vi "display_michelle_PKT_visjitter_stopadded_RandCont_PsuedoCO_TSLogFC2_forrecording.vi"() -> ()   [LabVIEW 2019]
uses:
  <vilib>/Analysis/Matrix/Datatypes/RealMatrix.ctl
  <vilib>/Utility/file.llb/Write Delimited Spreadsheet (DBL).vi
  <vilib>/Analysis/Matrix/NI_Matrix.lvlib
panel:
  out "lambda":dbl
  out "maxITI":dbl
  out "minITI":dbl
  out "goEXP":dbl
  out "meanITI":dbl
  out "Lag1":dbl
  out "TSLog":dbl[][](array[numeric])
  out "TSLog2":dbl[][](array[numeric])
  out "Initialtime":dbl
  out "Time Stamp":timestamp format="%<%H:%M:%S%4u>T"
  out "TSLog1":dbl[][](array[numeric])
  out "ArrayTemp3":T1
  out "StimID2":dbl
  out "Contrast":dbl
  out "TimeOutCounter":i32
  out "ElapsedTime_M":dbl
  out "Base_Contrast":dbl
  out "CurrentTrial":u32=1
  out "Jitter":dbl
  out "BaseITI":dbl
  out "VisStimDuration":dbl
  in  "Stop":bool
  out "Num trials":u32=204
  out "ISI Time":dbl
  out "Stim TS":dbl
  out "Output":dbl[][](array[numeric])
  out "Output frame":T1
  out "Array temp1":T1
  out "Elapsed Time":dbl
  out "Display":bool=TRUE
  out "Trial":u32=1
  out "reward":dbl[](array[numeric])
  out "stim_id":dbl[](array[numeric])
  out "stim_loaded":dbl
  out "Timings":dbl[](array[numeric])
  out "Stimuli Loaded?":bool
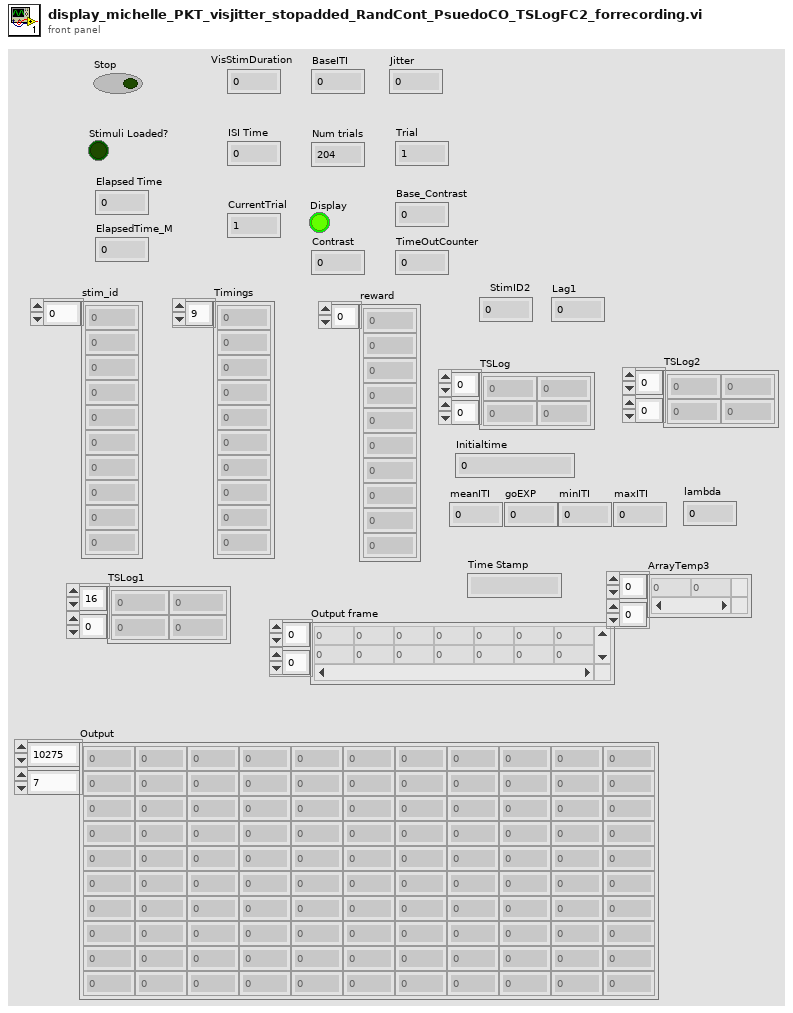
[diagram p1: front panel]
types:
  T1 = typedef "NI_Matrix.lvlib/RealMatrix.ctl" = dbl[][]
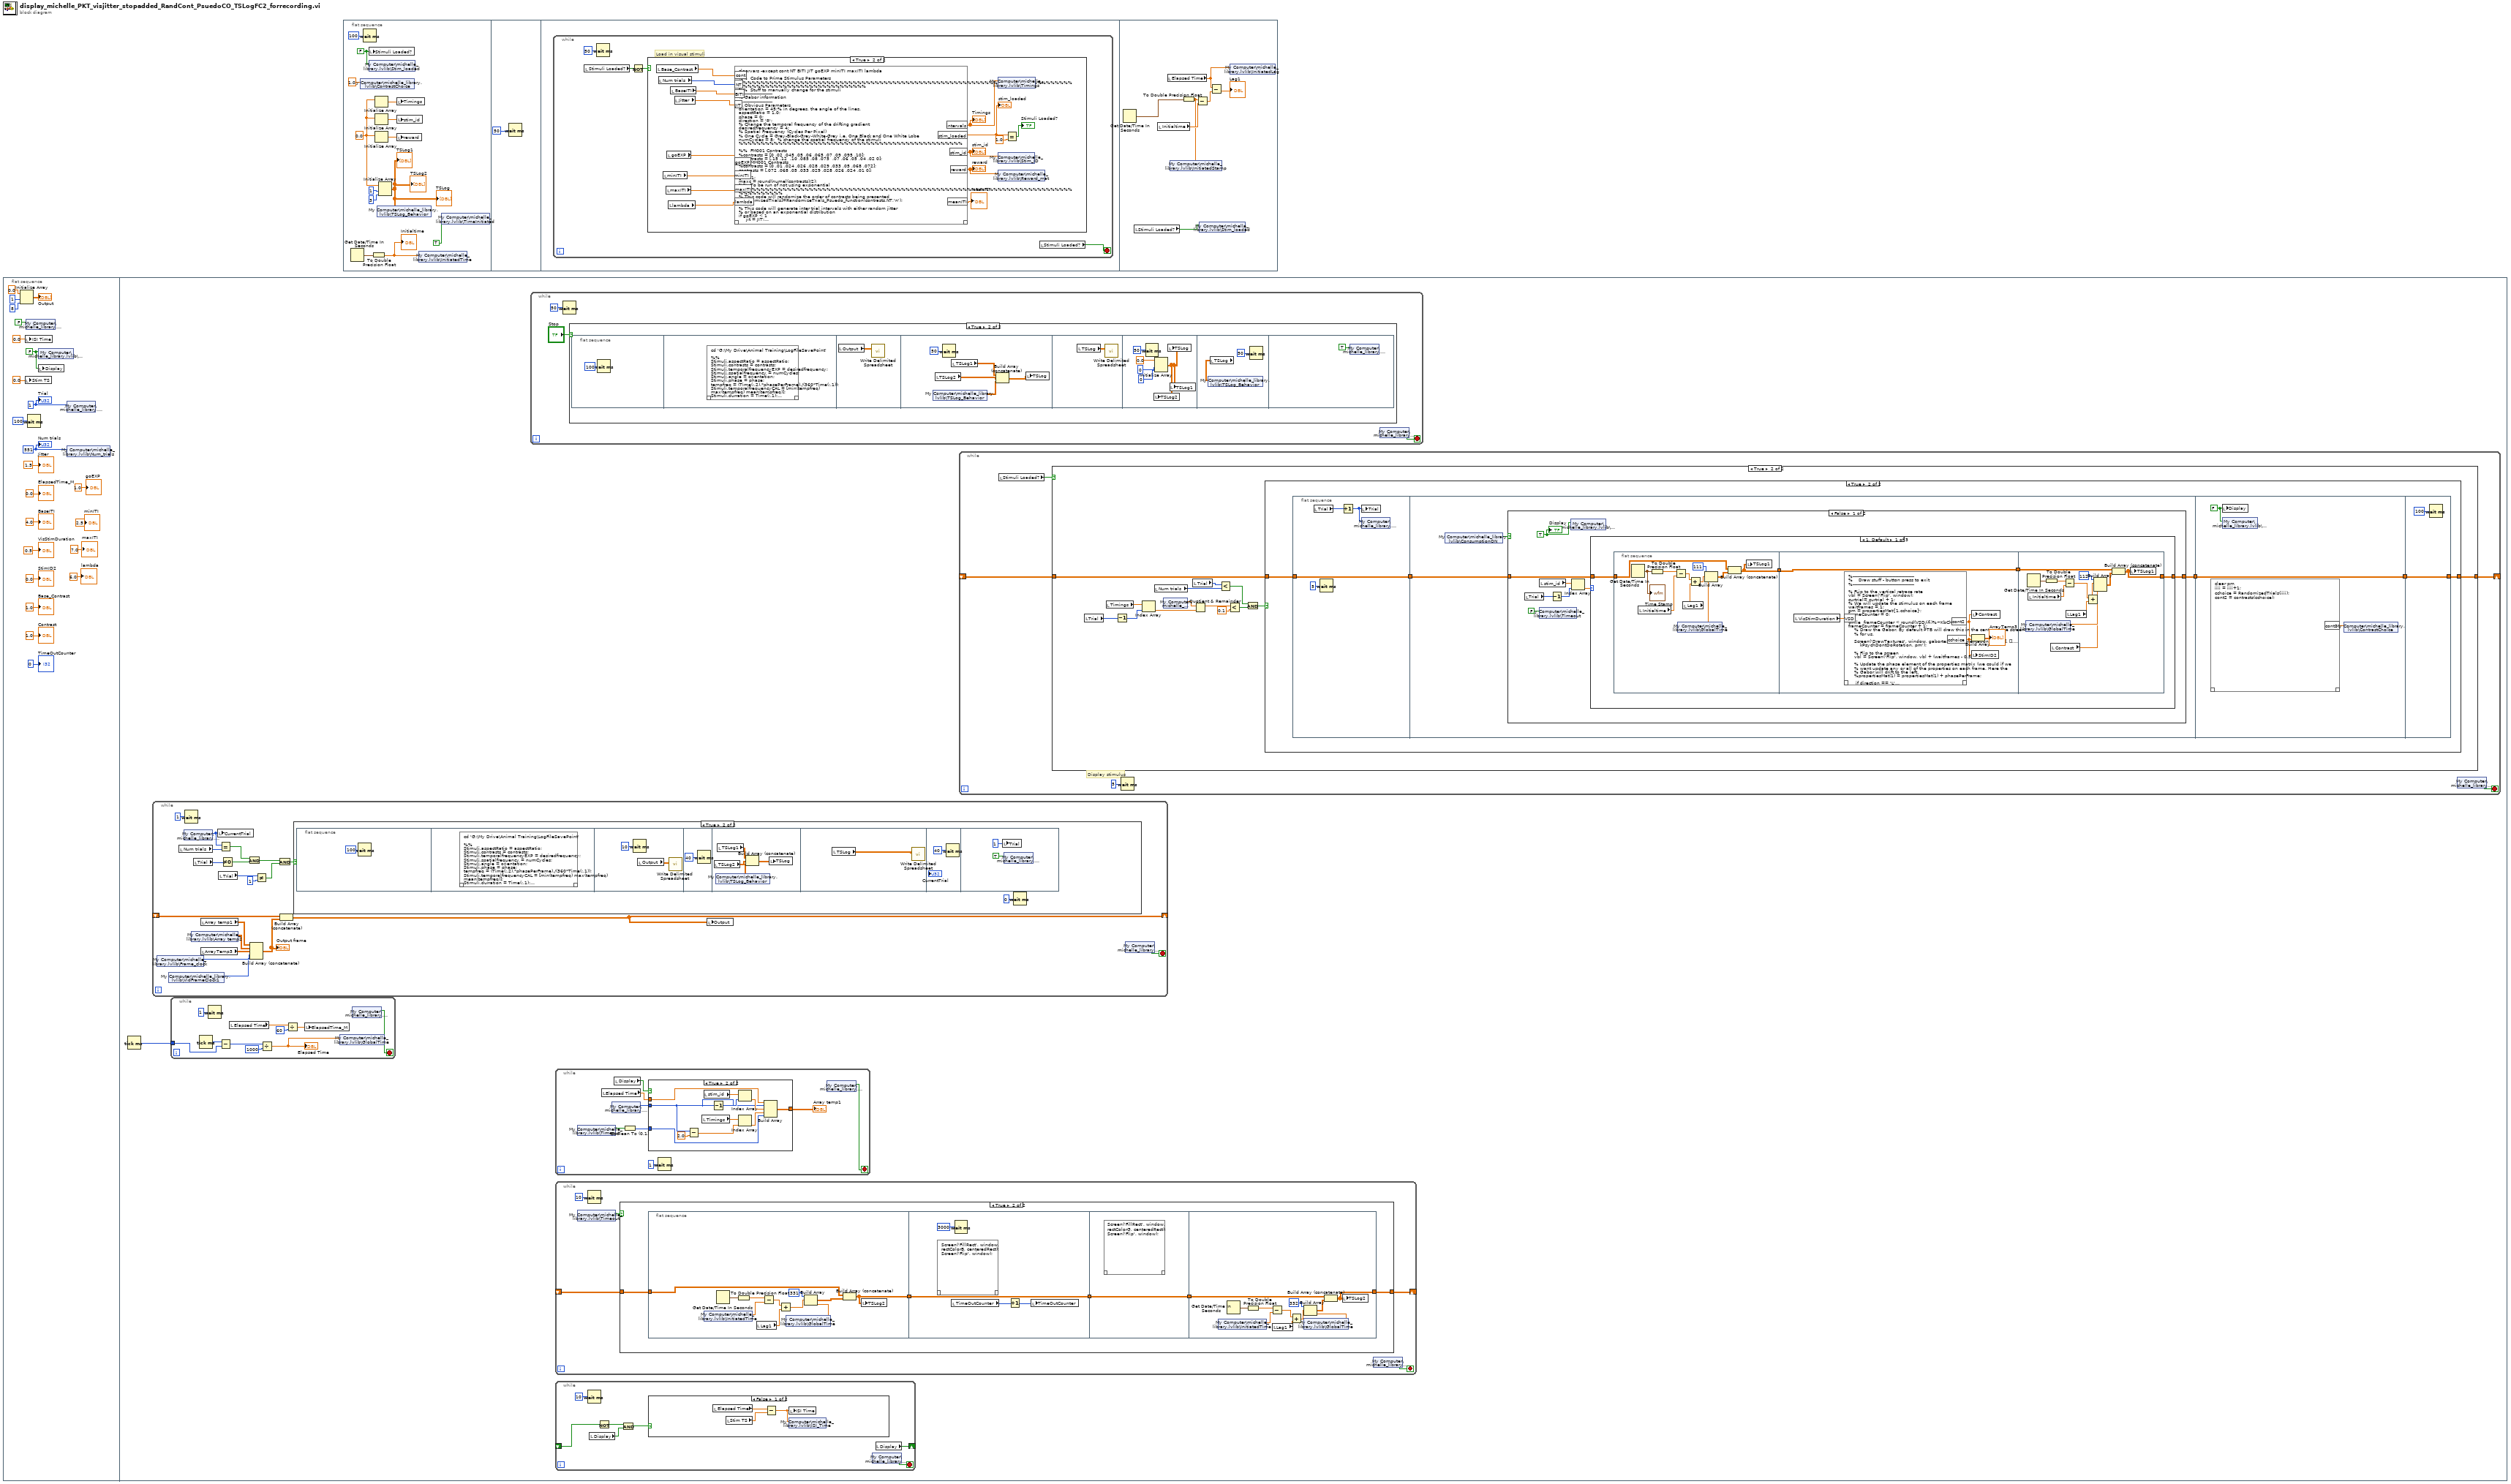
[diagram p0: block diagram]
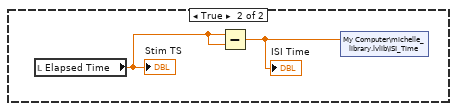
[diagram p5: hidden frame]
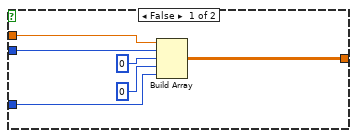
[diagram p6: hidden frame]
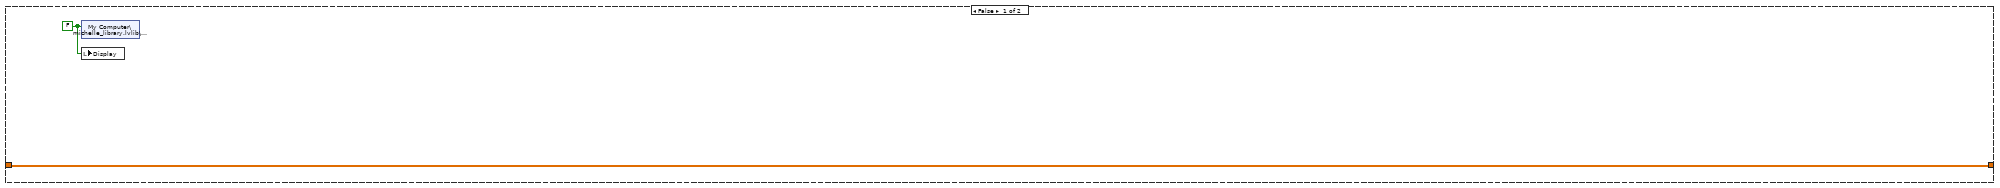
[diagram p9: hidden frame]
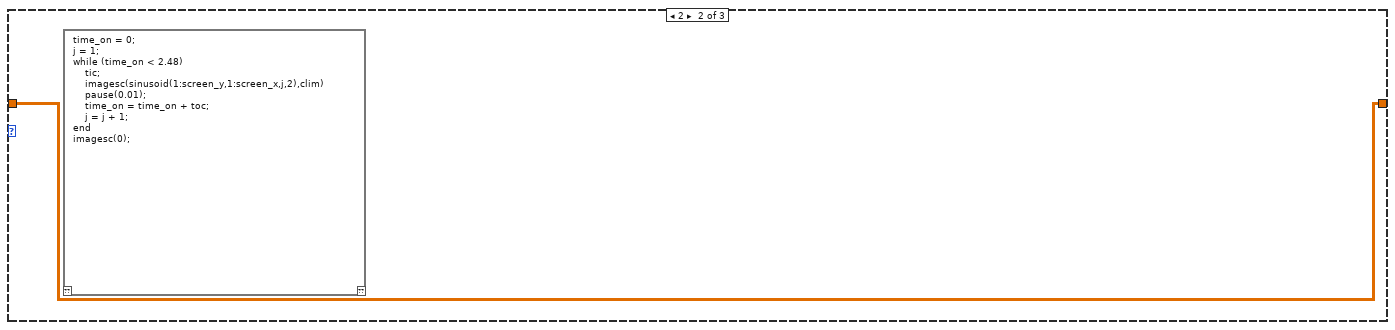
[diagram p10: hidden frame]
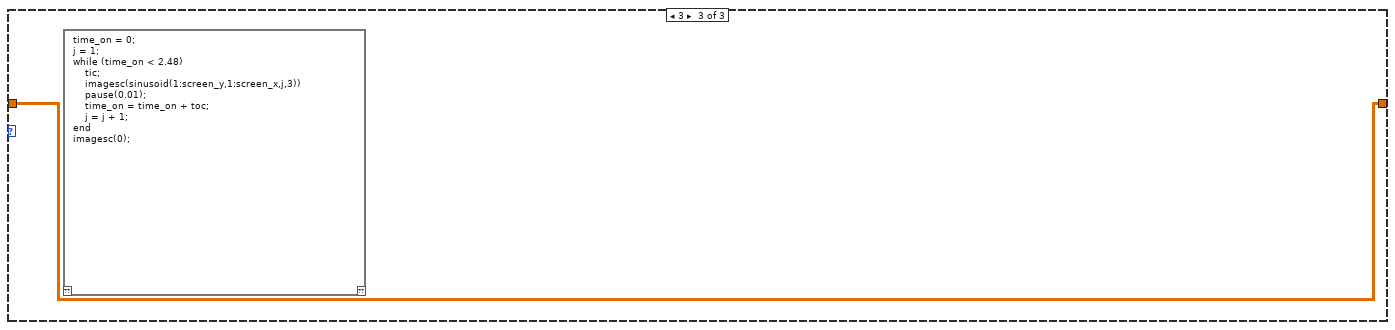
[diagram p11: hidden frame]
diagram:
  n1 = flat-sequence {
    frame #0 {
      w15 = u32 551
      w21 = FALSE ("Display")
      w23 = u32 1 ("Trial")
      n2 = Initialize Array(0.0 ("element"), 1 ("dimension size"), 8 ("dimension size")) -> (→"Output":dbl[][])
      n3 = local write "ISI Time"(0.0 ("ISI Time")) -> ()
      n4 = local write "Stim TS"(0.0 ("Stim TS")) -> ()
      n5 = shared-variable "My Computer\\michelle_library.lvlib\\Stop"(FALSE ("Stop")) -> ()  [unwired: 1 in, 1 out]
      n6 = Wait (ms)(milliseconds to wait=u32 100) -> ()  [unwired: 1 out]
      n7 = shared-variable "My Computer\\michelle_library.lvlib\\Display"(w21) -> ()  [unwired: 1 in, 1 out]
      n8 = local write "Display"(w21) -> ()
      n9 = shared-variable "My Computer\\michelle_library.lvlib\\Trial"(w23) -> ()  [unwired: 1 in, 1 out]
      n10 = shared-variable "My Computer\\michelle_library.lvlib\\Num_trials"(w15) -> ()  [unwired: 1 in, 1 out]
      "Trial" <- w23
      "Num trials" <- w15
      "VisStimDuration" <- 0.5
      "BaseITI" <- 4.0
      "Jitter" <- 1.5
      "Base_Contrast" <- 1.0
      "ElapsedTime_M" <- 0.0
      "TimeOutCounter" <- 0
      "Contrast" <- 1.0
      "StimID2" <- 0.0
      "goEXP" <- 1.0
      "minITI" <- 2.5
      "maxITI" <- 7.0
      "lambda" <- 6.0
    }
    frame #1 {
      n11 = Tick Count (ms)() -> (millisecond timer value=w24:u32)
      n12 = while {
        shift-right: [w145] -> _
        shift-left: _ -> [w146]
        stop <- w148 stop-if-true
        n13 = shared-variable "My Computer\\michelle_library.lvlib\\Frame_clock"() -> (w130:u32)  [unwired: 1 in, 1 out]
        n14 = shared-variable "My Computer\\michelle_library.lvlib\\VidFrameClock1"() -> (w129:u32)  [unwired: 1 in, 1 out]
        n15 = local read "Num trials"() -> (w141:u32)
        n16 = shared-variable "My Computer\\michelle_library.lvlib\\Trial"() -> (w132:u32)  [unwired: 1 in, 1 out]
        n17 = Wait (ms)(milliseconds to wait=u32 1) -> ()  [unwired: 1 out]
        n18 = shared-variable "My Computer\\michelle_library.lvlib\\Array temp2"() -> (w143:dbl[][])  [unwired: 1 in, 1 out]
        n19 = local read "Trial"() -> (w139:u32)
        n20 = local read "Array temp1"() -> (w144:T1)
        n21 = local read "ArrayTemp3"() -> (w131:T1)
        n22 = local write "CurrentTrial"(w132) -> ()
        n23 = local read "Trial"() -> (w138:u32)
        n24 = Equal?(x=w132, y=w141) -> (x = y?=w140:bool)
        n25 = Not Equal To 0?(x=w139) -> (x != 0?=w135:bool)
        n26 = And(x=w140, y=w135) -> (x .and. y?=w133:bool)
        n27 = Build Array (concatenate)(w144, w143, w131, w130, w129) -> (w142:T1)
        "Output frame" <- w142
        n28 = Not Equal?(x=w138, y=1) -> (x != y?=w137:bool)
        n29 = And(x=w133, y=w137) -> (x .and. y?=w134:bool)
        n30 = Build Array (concatenate) ("Build Matrix")(w146, w142) -> (w145:T1)
        n31 = case shown="True" w134 {
          frame False {
          }
          frame True {
            n32 = flat-sequence {
              frame #0 {
                n33 = Wait (ms)(milliseconds to wait=100) -> ()  [unwired: 1 out]
              }
              frame #1 {
                n34 = script code="cd 'G:\\My Drive\\Animal Training\\LogFileSavePoint'\n\n%%\nStimuli.aspectRatio = aspectRatio;\nStimuli.contrasts = contrasts;\nStimuli.temporalfrequencyEXP = desiredfrequency;\nStimuli.spatialfrequency = numCycles;\nStimuli.angle = orientation;\nStimuli.phase = phase;\ntempfreq = (Time(:,2).*phasePerFrame)./(360*Time(:,1)); \nStimuli.temporalfrequencyCAL = [min(tempfreq) max(tempfreq) mean(tempfreq)];\nStimuli.durration = Time(:,1);\nStimuli.frames = Time(:,2);\nStimuli.contrast = Time(:,3);\nStimuli.intervals = intervals;\nif goEXP == 0\n     int.type = 'jitter';\n     int.baseITI = BITI;\n     int.jitter = JIT;\nelseif goEXP == 1\n     int.type = 'exponential';\n     int.minITI = minITI;\n     int.maxITI = maxITI;\n     int.lambda = lambda;\nend\nStimuli.IntervalData = int;\n\n\nWindow.Xpixels = screenXpixels;\nWindow.Ypixels = screenYpixels;\nWindow.Xcenter = xCenter;\nWindow.Ycenter = yCenter;\nWindow.ifi = ifi;\nWindow.screen = screenNumber;\n\n%%\n[logname] = generatelogname();\n\nsave(logname,'Stimuli','Window');"() -> ()  [unwired: 1 in, 1 out]
              }
              frame #2 {
                n35 = Wait (ms)(milliseconds to wait=u32 10) -> ()  [unwired: 1 out]
                n36 = local read "Output"() -> (w152:dbl[][])
                n37 = call-poly <vilib>:"Write Delimited Spreadsheet.vi"("2D data"=w152) -> ()  [unwired: 13 in, 2 out]
              }
              frame #3 {
                n38 = Wait (ms)(milliseconds to wait=u32 40) -> ()  [unwired: 1 out]
              }
              frame #4 {
                n39 = local read "TSLog2"() -> (w157:dbl[][])
                n40 = shared-variable "My Computer\\michelle_library.lvlib\\TSLog_Behavior"() -> (w155:dbl[][])  [unwired: 1 in, 1 out]
                n41 = local read "TSLog1"() -> (w156:dbl[][])
                n42 = Build Array (concatenate) ("Build Matrix")(w156, w157, w155) -> (w154:T1)
                n43 = local write "TSLog"(w154) -> ()
              }
              frame #5 {
                n44 = local read "TSLog"() -> (w158:dbl[][])
                n45 = call-poly <vilib>:"Write Delimited Spreadsheet.vi"("2D data"=w158) -> ()  [unwired: 13 in, 2 out]
              }
              frame #6 {
                n46 = Wait (ms)(milliseconds to wait=u32 40) -> ()  [unwired: 1 out]
              }
              frame #7 {
                n47 = local write "Trial"(1) -> ()
                n48 = shared-variable "My Computer\\michelle_library.lvlib\\Stop"(TRUE) -> ()  [unwired: 1 in, 1 out]
              }
            }
            n49 = Wait (ms)(milliseconds to wait=0) -> ()  [unwired: 1 out]
          }
        }
        n50 = local write "Output"(w145) -> ()
        n51 = shared-variable "My Computer\\michelle_library.lvlib\\Stop"() -> (w148:bool)  [unwired: 1 in, 1 out]
      }
      n52 = while {
        tunnel: w24 -> [w126]
        stop <- w123 stop-if-true
        n53 = Tick Count (ms)() -> (millisecond timer value=w127:u32)
        n54 = Wait (ms)(milliseconds to wait=u32 1) -> ()  [unwired: 1 out]
        n55 = Subtract(x=w127, y=w126) -> (x-y=w124:u32)
        n56 = local read "Elapsed Time"() -> (w121:dbl)
        n57 = Divide(x=w124, y=u32 1000) -> (x/y=w119:dbl)
        "Elapsed Time" <- w119
        n58 = Divide(x=w121, y=60) -> (x/y=w120:dbl)
        n59 = local write "ElapsedTime_M"(w120) -> ()
        n60 = shared-variable "My Computer\\michelle_library.lvlib\\GlobalTime"(w119) -> ()  [unwired: 1 in, 1 out]
        n61 = shared-variable "My Computer\\michelle_library.lvlib\\Stop"() -> (w123:bool)  [unwired: 1 in, 1 out]
      }
      n62 = while {
        stop <- w27 stop-if-true
        n63 = Wait (ms)(milliseconds to wait=50) -> ()  [unwired: 1 out]
        n64 = case shown="True" "Stop" {
          frame False {
          }
          frame True {
            n65 = flat-sequence {
              frame #0 {
                n66 = Wait (ms)(milliseconds to wait=100) -> ()  [unwired: 1 out]
              }
              frame #1 {
                n67 = script code="cd 'G:\\My Drive\\Animal Training\\LogFileSavePoint'\n\n%%\nStimuli.aspectRatio = aspectRatio;\nStimuli.contrasts = contrasts;\nStimuli.temporalfrequencyEXP = desiredfrequency;\nStimuli.spatialfrequency = numCycles;\nStimuli.angle = orientation;\nStimuli.phase = phase;\ntempfreq = (Time(:,2).*phasePerFrame)./(360*Time(:,1)); \nStimuli.temporalfrequencyCAL = [min(tempfreq) max(tempfreq) mean(tempfreq)];\nStimuli.durration = Time(:,1);\nStimuli.frames = Time(:,2);\nStimuli.contrast = Time(:,3);\nStimuli.intervals = intervals;\nif goEXP == 0\n     int.type = 'jitter';\n     int.baseITI = BITI;\n     int.jitter = JIT;\nelseif goEXP == 1\n     int.type = 'exponential';\n     int.minITI = minITI;\n     int.maxITI = maxITI;\n     int.lambda = lambda;\nend\nStimuli.IntervalData = int;\n\n\nWindow.Xpixels = screenXpixels;\nWindow.Ypixels = screenYpixels;\nWindow.Xcenter = xCenter;\nWindow.Ycenter = yCenter;\nWindow.ifi = ifi;\nWindow.screen = screenNumber;\n\n%%\n[logname] = generatelogname();\n\nsave(logname,'Stimuli','Window');"() -> ()  [unwired: 1 in, 1 out]
              }
              frame #2 {
                n68 = local read "Output"() -> (w29:dbl[][])
                n69 = call-poly <vilib>:"Write Delimited Spreadsheet.vi"("2D data"=w29) -> ()  [unwired: 13 in, 2 out]
              }
              frame #3 {
                n70 = shared-variable "My Computer\\michelle_library.lvlib\\TSLog_Behavior"() -> (w30:dbl[][])  [unwired: 1 in, 1 out]
                n71 = local read "TSLog2"() -> (w33:dbl[][])
                n72 = Wait (ms)(milliseconds to wait=50) -> ()  [unwired: 1 out]
                n73 = local read "TSLog1"() -> (w32:dbl[][])
                n74 = Build Array (concatenate) ("Build Matrix")(w32, w33, w30) -> (w31:T1)
                n75 = local write "TSLog"(w31) -> ()
              }
              frame #4 {
                n76 = local read "TSLog"() -> (w35:dbl[][])
                n77 = call-poly <vilib>:"Write Delimited Spreadsheet.vi"("2D data"=w35) -> ()  [unwired: 13 in, 2 out]
              }
              frame #5 {
                n78 = Wait (ms)(milliseconds to wait=50) -> ()  [unwired: 1 out]
                n79 = Initialize Array(0.0, 0, 0) -> (w37:dbl[][])
                n80 = local write "TSLog2"(w37) -> ()
                n81 = local write "TSLog"(w37) -> ()
                n82 = local write "TSLog1"(w37) -> ()
              }
              frame #6 {
                n83 = local read "TSLog"() -> (w42:dbl[][])
                n84 = shared-variable "My Computer\\michelle_library.lvlib\\TSLog_Behavior"(w42) -> ()  [unwired: 1 in, 1 out]
                n85 = Wait (ms)(milliseconds to wait=50) -> ()  [unwired: 1 out]
              }
              frame #7 {
                n86 = shared-variable "My Computer\\michelle_library.lvlib\\Stop"(TRUE) -> ()  [unwired: 1 in, 1 out]
              }
            }
          }
        }
        n87 = shared-variable "My Computer\\michelle_library.lvlib\\Stop"() -> (w27:bool)  [unwired: 1 in, 1 out]
      }
      n88 = while {
        stop <- w96 stop-if-true
        n89 = shared-variable "My Computer\\michelle_library.lvlib\\Timeout"() -> (w94:bool)  [unwired: 1 in, 1 out]
        n90 = local read "Elapsed Time"() -> (w100:dbl)
        n91 = shared-variable "My Computer\\michelle_library.lvlib\\Trial"() -> (w98:u32)  [unwired: 1 in, 1 out]
        n92 = local read "Display"() -> (w97:bool)
        n93 = Boolean To (0,1)(Boolean=w94) -> (0, 1=w95:i16)
        n94 = case shown="True" w97 {
          tunnel: w98 -> [w106 w109]
          tunnel: w100 -> [w107 w116]
          tunnel: [w105 w117] -> w99
          tunnel: w95 -> [w102 w111]
          frame False {
            n95 = Build Array(w107, w106, u32 0 ("milliseconds to wait"), 0, w102) -> (w105:T1)
          }
          frame True {
            n96 = Subtract(x=w109, y=2.0) -> (x-y=w108:dbl)
            n97 = local read "Timings"() -> (w114:dbl[])
            n98 = local read "stim_id"() -> (w118:dbl[])
            n99 = Decrement(x=w109) -> (x-1=w113:u32)
            n100 = Index Array(array=w118, index=w113) -> (element=w115:dbl)
            n101 = Index Array(array=w114, index=w108) -> (element=w112:dbl)
            n102 = Build Array(w116, w109, w115, w112, w111) -> (w117:T1)
          }
        }
        "Array temp1" <- w99
        n103 = Wait (ms)(milliseconds to wait=u32 1) -> ()  [unwired: 1 out]
        n104 = shared-variable "My Computer\\michelle_library.lvlib\\Stop"() -> (w96:bool)  [unwired: 1 in, 1 out]
      }
      n105 = while {
        shift-right: [w44] -> _
        shift-left: _ -> [w45]
        stop <- w48 stop-if-true
        n106 = shared-variable "My Computer\\michelle_library.lvlib\\Timeout"() -> (w46:bool)  [unwired: 1 in, 1 out]
        n107 = Wait (ms)(milliseconds to wait=u32 10) -> ()  [unwired: 1 out]
        n108 = case shown="True" w46 {
          tunnel: w45 -> [w49 w54]
          tunnel: [w49 w53] -> w44
          frame False {
          }
          frame True {
            n109 = flat-sequence {
              tunnel: w54 -> [w60]
              tunnel: [w59] -> w51
              tunnel: [w66] -> w52
              tunnel: w51 -> [w66]
              tunnel: w52 -> [w70]
              tunnel: [w70] -> w50
              tunnel: [w75] -> w53
              tunnel: w50 -> [w76]
              frame #0 {
                n110 = shared-variable "My Computer\\michelle_library.lvlib\\InitiatedTime"() -> (w63:dbl)  [unwired: 1 in, 1 out]
                n111 = Get Date/Time In Seconds() -> (seconds since 1Jan1904=w65:timestamp)
                n112 = To Double Precision Float(number=w65) -> (double precision float=w64:dbl)
                n113 = local read "Lag1"() -> (w56:dbl)
                n114 = Subtract(x=w64, y=w63) -> (x-y=w57:dbl)
                n115 = Add(x=w57, y=w56) -> (x+y=w58:dbl)
                n116 = shared-variable "My Computer\\michelle_library.lvlib\\GlobalTime"() -> (w55:dbl)  [unwired: 1 in, 1 out]
                n117 = Build Array(331, w58, w55) -> (w62:T1)
                n118 = Build Array (concatenate) ("Build Matrix")(w60, w62) -> (w59:T1)
                n119 = local write "TSLog2"(w59) -> ()
              }
              frame #1 {
                n120 = script code="Screen('FillRect', window, rectColorB, centeredRect);\nScreen('Flip', window);"() -> ()  [unwired: 1 in, 1 out]
                n121 = local read "TimeOutCounter"() -> (w68:i32)
                n122 = Wait (ms)(milliseconds to wait=u32 3000) -> ()  [unwired: 1 out]
                n123 = Increment(x=w68) -> (x+1=w67:i32)
                n124 = local write "TimeOutCounter"(w67) -> ()
              }
              frame #2 {
                n125 = script code="Screen('FillRect', window, rectColorG, centeredRect);\nScreen('Flip', window);"() -> ()  [unwired: 1 in, 1 out]
              }
              frame #3 {
                n126 = shared-variable "My Computer\\michelle_library.lvlib\\InitiatedTime"() -> (w81:dbl)  [unwired: 1 in, 1 out]
                n127 = Get Date/Time In Seconds() -> (seconds since 1Jan1904=w79:timestamp)
                n128 = To Double Precision Float(number=w79) -> (double precision float=w80:dbl)
                n129 = Subtract(x=w80, y=w81) -> (x-y=w73:dbl)
                n130 = local read "Lag1"() -> (w72:dbl)
                n131 = Add(x=w73, y=w72) -> (x+y=w74:dbl)
                n132 = shared-variable "My Computer\\michelle_library.lvlib\\GlobalTime"() -> (w71:dbl)  [unwired: 1 in, 1 out]
                n133 = Build Array(332, w74, w71) -> (w77:T1)
                n134 = Build Array (concatenate) ("Build Matrix")(w76, w77) -> (w75:T1)
                n135 = local write "TSLog2"(w75) -> ()
              }
            }
          }
        }
        n136 = shared-variable "My Computer\\michelle_library.lvlib\\Stop"() -> (w48:bool)  [unwired: 1 in, 1 out]
      }
      n137 = while {
        shift-right: [w86] -> _
        shift-left: _ -> [w85]
        stop <- w88 stop-if-true
        n138 = Wait (ms)(milliseconds to wait=u32 10) -> ()  [unwired: 1 out]
        n139 = local read "Display"() -> (w83:bool)
        n140 = Not(x=w85) -> (.not. x?=w84:bool)
        n141 = And(x=w84, y=w83) -> (x .and. y?=w82:bool)
        n142 = case shown="False" w82 {
          frame False {
            n143 = local read "Elapsed Time"() -> (w89:dbl)
            n144 = local read "Stim TS"() -> (w91:dbl)
            n145 = Subtract(x=w89, y=w91) -> (x-y=w90:dbl)
            n146 = local write "ISI Time"(w90) -> ()
            n147 = shared-variable "My Computer\\michelle_library.lvlib\\ISI_Time"(w90) -> ()  [unwired: 1 in, 1 out]
          }
          frame True {
            n148 = local read "Elapsed Time"() -> (w92:dbl)
            "Stim TS" <- w92
            n149 = Subtract(x=w92, y=w92) -> (x-y=w93:dbl)
            "ISI Time" <- w93
            n150 = shared-variable "My Computer\\michelle_library.lvlib\\ISI_Time"(w93) -> ()  [unwired: 1 in, 1 out]
          }
        }
        n151 = shared-variable "My Computer\\michelle_library.lvlib\\Stop"() -> (w88:bool)  [unwired: 1 in, 1 out]
        n152 = local read "Display"() -> (w86:bool)
      }
      n153 = while {
        shift-right: [w162] -> _
        shift-left: _ -> [w163]
        stop <- w165 stop-if-true
        # "Display stimulus"
        n154 = local read "Stimuli Loaded?"() -> (w164:bool)
        n155 = case shown="True" w164 {
          tunnel: w163 -> [w167 w169]
          tunnel: [w167 w168] -> w162
          frame False {
          }
          frame True {
            n156 = local read "Trial"() -> (w170:u32)
            n157 = local read "Timings"() -> (w179:dbl[])
            n158 = Decrement(x=w170) -> (x-1=w171:u32)
            n159 = Index Array(array=w179, index=w171) -> (element=w178:dbl)
            n160 = local read "Num trials"() -> (w174:u32)
            n161 = shared-variable "My Computer\\michelle_library.lvlib\\ISI"() -> (w173:dbl)  [unwired: 1 in, 1 out]
            n162 = local read "Trial"() -> (w177:u32)
            n163 = Quotient & Remainder(x=w173, y=w178) -> (x-y*floor(x/y)=w181:dbl)  [unwired: 1 out]
            n164 = Less?(x=w177, y=w174) -> (x < y?=w176:bool)
            n165 = Less?(x=w181, y=0.1) -> (x < y?=w175:bool)
            n166 = And(x=w176, y=w175) -> (x .and. y?=w172:bool)
            n167 = case shown="True" w172 {
              tunnel: w169 -> [w182 w187]
              tunnel: [w182 w186] -> w168
              frame False {
                w183 = FALSE ("Display")
                n168 = shared-variable "My Computer\\michelle_library.lvlib\\Display"(w183) -> ()  [unwired: 1 in, 1 out]
                n169 = local write "Display"(w183) -> ()
              }
              frame True {
                n170 = flat-sequence {
                  tunnel: [w189] -> w188
                  tunnel: w187 -> [w189]
                  tunnel: w188 -> [w194]
                  tunnel: [w193] -> w184
                  tunnel: [w239] -> w185
                  tunnel: w184 -> [w239]
                  tunnel: [w242] -> w186
                  tunnel: w185 -> [w242]
                  frame #0 {
                    n171 = local read "Trial"() -> (w192:u32)
                    n172 = Wait (ms)(milliseconds to wait=u32 5) -> ()  [unwired: 1 out]
                    n173 = Increment(x=w192) -> (x+1=w191:u32)
                    n174 = local write "Trial"(w191) -> ()
                    n175 = shared-variable "My Computer\\michelle_library.lvlib\\Trial"(w191) -> ()  [unwired: 1 in, 1 out]
                  }
                  frame #1 {
                    n176 = shared-variable "My Computer\\michelle_library.lvlib\\ConsumptionON"() -> (w195:bool)  [unwired: 1 in, 1 out]
                    n177 = case shown="False" w195 {
                      tunnel: w194 -> [w197 w238]
                      tunnel: [w196 w238] -> w193
                      frame False {
                        w198 = TRUE ("Boolean")
                        n178 = local read "Trial"() -> (w201:u32)
                        n179 = shared-variable "My Computer\\michelle_library.lvlib\\Timeout"(FALSE) -> ()  [unwired: 1 in, 1 out]
                        n180 = local read "stim_id"() -> (w203:dbl[])
                        n181 = Decrement(x=w201) -> (x-1=w200:u32)
                        n182 = shared-variable "My Computer\\michelle_library.lvlib\\Display"(w198) -> ()  [unwired: 1 in, 1 out]
                        n183 = Index Array(array=w203, index=w200) -> (element=w202:dbl)
                        n184 = case shown="1, Default" w202 {
                          tunnel: w197 -> [w207 w236 w237]
                          tunnel: [w206 w236 w237] -> w196
                          frame 1, Default {
                            n185 = flat-sequence {
                              tunnel: w207 -> [w217]
                              tunnel: [w216] -> w205
                              tunnel: w205 -> [w219]
                              tunnel: [w219] -> w204
                              tunnel: [w234] -> w206
                              tunnel: w204 -> [w233]
                              frame #0 {
                                n186 = Get Date/Time In Seconds() -> (seconds since 1Jan1904=w214:timestamp)
                                "Time Stamp" <- w214
                                n187 = local read "Initialtime"() -> (w212:dbl)
                                n188 = To Double Precision Float(number=w214) -> (double precision float=w213:dbl)
                                n189 = Subtract(x=w213, y=w212) -> (x-y=w210:dbl)
                                n190 = shared-variable "My Computer\\michelle_library.lvlib\\GlobalTime"() -> (w208:dbl)  [unwired: 1 in, 1 out]
                                n191 = local read "Lag1"() -> (w211:dbl)
                                n192 = Add(x=w210, y=w211) -> (x+y=w209:dbl)
                                n193 = Build Array(111, w209, w208) -> (w215:T1)
                                n194 = Build Array (concatenate) ("Build Matrix")(w217, w215) -> (w216:T1)
                                n195 = local write "TSLog1"(w216) -> ()
                              }
                              frame #1 {
                                n196 = local read "VisStimDuration"() -> (w221:dbl)
                                n197 = script code="%------------------------------------------\n%    Draw stuff - button press to exit\n%------------------------------------------\n\n% FLip to the vertical retrace rate\nvbl = Screen('Flip', window);\ncurtrial= curtrial + 1;\n% We will update the stimulus on each frame\nwaitframes = 1;\npm = propertiesMat{1,cchoice};\nframeCounter = 0;\ntic\nwhile  frameCounter < round(VSD/ifi)%~KbCheck\nframeCounter = frameCounter + 1;\n    % Draw the Gabor. By default PTB will draw this in the center of the screen\n    % for us.\n   \n    Screen('DrawTextures', window, gabortex, [], [], orientation, [], [], [], [],...\n        kPsychDontDoRotation, pm');\n\n    % Flip to the screen\n    vbl = Screen('Flip', window, vbl + (waitframes - 0.5) * ifi);\n\n    % Update the phase element of the properties matrix (we could if we\n    % want update any or all of the properties on each frame. Here the\n    % Gabor will drift to the left.\n    %propertiesMat(1) = propertiesMat(1) + phasePerFrame;\n \n     if direction == 'L'\n          pm(1) = pm(1) + phasePerFrame;\n     elseif direction =='R'\n          pm(1) = pm(1) - phasePerFrame;\n     end\n\nend\nTime(curtrial,1) = toc;\nTime(curtrial,2) = frameCounter;\nTime(curtrial,3) = pm(4);\nvbl = Screen('Flip', window);"("VSD"=w221) -> ("cont2"=w223:dbl, "cchoice"=w222:dbl)  [unwired: 1 in, 1 out]
                                n198 = local write "Contrast"(w223) -> ()
                                n199 = Build Array(w223, w222) -> (→"ArrayTemp3":T1)
                                n200 = local write "StimID2"(w222) -> ()
                              }
                              frame #2 {
                                n201 = shared-variable "My Computer\\michelle_library.lvlib\\GlobalTime"() -> (w225:dbl)  [unwired: 1 in, 1 out]
                                n202 = Get Date/Time In Seconds() -> (seconds since 1Jan1904=w231:timestamp)
                                n203 = local read "Initialtime"() -> (w230:dbl)
                                n204 = To Double Precision Float(number=w231) -> (double precision float=w229:dbl)
                                n205 = local read "Contrast"() -> (w224:dbl)
                                n206 = Subtract(x=w229, y=w230) -> (x-y=w228:dbl)
                                n207 = local read "Lag1"() -> (w226:dbl)
                                n208 = Add(x=w228, y=w226) -> (x+y=w227:dbl)
                                n209 = Build Array(112, w227, w225, w224) -> (w235:T1)
                                n210 = Build Array (concatenate) ("Build Matrix")(w233, w235) -> (w234:T1)
                                n211 = local write "TSLog1"(w234) -> ()
                              }
                            }
                          }
                          frame 2 {
                            n212 = script code="time_on = 0;\nj = 1;\nwhile (time_on < 2.48)\n    tic;\n    imagesc(sinusoid(1:screen_y,1:screen_x,j,2),clim)\n    pause(0.01);\n    time_on = time_on + toc;\n    j = j + 1;\nend\nimagesc(0);"() -> ()  [unwired: 1 in, 1 out]
                          }
                          frame 3 {
                            n213 = script code="time_on = 0;\nj = 1;\nwhile (time_on < 2.48)\n    tic;\n    imagesc(sinusoid(1:screen_y,1:screen_x,j,3))\n    pause(0.01);\n    time_on = time_on + toc;\n    j = j + 1;\nend\nimagesc(0);"() -> ()  [unwired: 1 in, 1 out]
                          }
                        }
                        "Display" <- w198
                      }
                      frame True {
                      }
                    }
                  }
                  frame #2 {
                    w241 = FALSE ("Display")
                    n214 = script code="clear pm\niiii = iiii+1;\ncchoice = RandomizedTrials(iiii);\ncont2 = contrasts(cchoice);"() -> ("cont2"=w240:dbl)  [unwired: 1 in, 1 out]
                    n215 = local write "Display"(w241) -> ()
                    n216 = shared-variable "My Computer\\michelle_library.lvlib\\Display"(w241) -> ()  [unwired: 1 in, 1 out]
                    n217 = shared-variable "My Computer\\michelle_library.lvlib\\ContrastChoice"(w240) -> ()  [unwired: 1 in, 1 out]
                  }
                  frame #3 {
                    n218 = Wait (ms)(milliseconds to wait=u32 100) -> ()  [unwired: 1 out]
                  }
                }
              }
            }
          }
        }
        n219 = Wait (ms)(milliseconds to wait=u32 5) -> ()  [unwired: 1 out]
        n220 = shared-variable "My Computer\\michelle_library.lvlib\\Stop"() -> (w165:bool)  [unwired: 1 in, 1 out]
      }
    }
  }
  n221 = flat-sequence {
    frame #0 {
      w250 = 0.0 ("element")
      w252 = FALSE ("Stimuli Loaded?")
      n222 = Get Date/Time In Seconds() -> (seconds since 1Jan1904=w247:timestamp)
      n223 = shared-variable "My Computer\\michelle_library.lvlib\\ContrastChoice"(1.0) -> ()  [unwired: 1 in, 1 out]
      n224 = Wait (ms)(milliseconds to wait=u32 100) -> ()  [unwired: 1 out]
      n225 = local write "Stimuli Loaded?"(w252) -> ()
      n226 = shared-variable "My Computer\\michelle_library.lvlib\\Stim_loaded"(w252) -> ()  [unwired: 1 in, 1 out]
      n227 = To Double Precision Float(number=w247) -> (double precision float=w246:dbl)
      "Initialtime" <- w246
      n228 = Initialize Array(w250) -> (w255:dbl[])  [unwired: 1 in]
      n229 = Initialize Array(w250) -> (w254:dbl[])  [unwired: 1 in]
      n230 = Initialize Array(w250) -> (w253:dbl[])  [unwired: 1 in]
      n231 = Initialize Array(w250, 1, 3) -> (w244:dbl[][])
      "TSLog1" <- w244
      "TSLog2" <- w244
      "TSLog" <- w244
      n232 = shared-variable "My Computer\\michelle_library.lvlib\\TSLog_Behavior"(w244) -> ()  [unwired: 1 in, 1 out]
      n233 = local write "Timings"(w255) -> ()
      n234 = local write "stim_id"(w254) -> ()
      n235 = local write "reward"(w253) -> ()
      n236 = shared-variable "My Computer\\michelle_library.lvlib\\InitiatedTime"(w246) -> ()  [unwired: 1 in, 1 out]
      n237 = shared-variable "My Computer\\michelle_library.lvlib\\TimeInitiated"(TRUE) -> ()  [unwired: 1 in, 1 out]
    }
    frame #1 {
      n238 = Wait (ms)(milliseconds to wait=u32 50) -> ()  [unwired: 1 out]
    }
    frame #2 {
      n239 = while {
        stop <- w258 stop-if-true
        # "Load in visual stimuli"
        n240 = local read "Stimuli Loaded?"() -> (w260:bool)
        n241 = Wait (ms)(milliseconds to wait=u32 50) -> ()  [unwired: 1 out]
        n242 = Not(x=w260) -> (.not. x?=w259:bool)
        n243 = case shown="True" w259 {
          frame False {
          }
          frame True {
            n244 = local read "Base_Contrast"() -> (w268:dbl)
            n245 = local read "Num trials"() -> (w271:u32)
            n246 = local read "minITI"() -> (w264:dbl)
            n247 = local read "maxITI"() -> (w263:dbl)
            n248 = local read "goEXP"() -> (w265:dbl)
            n249 = local read "lambda"() -> (w262:dbl)
            n250 = local read "BaseITI"() -> (w270:dbl)
            n251 = local read "Jitter"() -> (w269:dbl)
            n252 = script code="clearvars -except cont NT BITI JIT goEXP minITI maxITI lambda\n\n%%  Code to Prime Stimulus Parameters\n%%%%%%%%%%%%%%%%%%%%%%%%%%%%%%%%%%%%%%%%%%%%%%%%%%%%%%%%%%%%%%%%%%%%%%%%%%%%%%%%%%%%%%%%%%%%%%%%%%%%%%%%%\n%%  Stuff to manually change for the stimuli\n%--------------------\n% Gabor information\n%--------------------\n% Obvious Parameters\norientation = 45;% in degrees, the angle of the lines.\naspectRatio = 1.0;\nphase = 0;\ndirection = 'R';\n% Change the temporal frequency of the drifting gradient\ndesiredfrequency = 4;\n% Spatial Frequency (Cycles Per Pixel)\n% One Cycle = Grey-Black-Grey-White-Grey i.e. One Black and One White Lobe\nnumCycles = 8;  % change the spatial frequency of the stimuli\n%%%%%%%%%%%%%%%%%%%%%%%%%%%%%%%%%%%%%%%%%%%%%%%%%%%\n\n%%  FM001 Contrasts\n%contrasts = [0 .02 .045 .05 .06 .065 .07 .09 .095 .10];\n%contrasts = [.15 .12  .10 .085 .08 .075  .07 .06 .05 .04 .02 0];\n%%  MM001 Contrasts\n%contrasts = [0 .01 .024 .026 .028 .029 .033 .05 .068 .072];\ncontrasts = [.072 .068 .05 .033 .029 .028 .026 .024 .01 0];\n\ngo = 1;\nmaxc = round(numel(contrasts)/2);\n%%  To be run of not using exponential\n%%%%%%%%%%%%%%%%%%%%%%%%%%%%%%%%%%%%%%%%%%%%%%%%%%%%%%%%%%%%%%%%%%%%%%%%%%%%%%%%%%%%%%\n% This code will randomize the order of contrasts being presented\n[RandomizedTrials]=RandomizeTrials_Psuedo_function(contrasts,NT,'n');\n\n% This code will generate inter trial intervals with either random jitter\n% or based on an exponential distribution\nif goEXP < 1\n     jit = JIT;\n     jitter = rand(1,NT);\n     jitter = 2*jit*(jitter- .5);\n     ITIbase = BITI;\n     intervals = [ones(1,NT)*ITIbase];\n     intervals = intervals + jitter;\nelseif goEXP > 0\n     intervals = exponentialITI(1/lambda, minITI, maxITI, NT);\nend\n\n%%  Prep the stimulus presentation software\n%%%%%%%%%%%%%%%%%%%%%%%%%%%%%%%%%%%%%%%%%%%%%%%%%%%%%%%%%%%%%%%%%%%%%%%%%%%\nScreen('Preference', 'SkipSyncTests', 1);\nsca;\nclose all;\n% Setup PTB with some default values\nPsychDefaultSetup(2);\n% Set the screen number to the external secondary monitor if there is one connected\nscreenNumber = max(Screen('Screens'));\n\n% Define black, white and grey\nwhite = WhiteIndex(screenNumber);\nblack = BlackIndex(screenNumber);\ngrey = white / 2;\n\n% Open the screen & define it's dimensions\n[window, windowRect] = PsychImaging('OpenWindow', screenNumber, grey,...\n    [], 32, 2, [], [], kPsychNeedRetinaResolution);\n[screenXpixels, screenYpixels] = Screen('WindowSize', window);\n[xCenter, yCenter] = RectCenter(windowRect);\n\n% Get the vertical refresh rate of the monitor\nifi = Screen('GetFlipInterval', window);\n\n% Set maximum priority level\ntopPriorityLevel = MaxPriority(window);\nPriority(topPriorityLevel);\n\n\n% Build a procedural gabor texture (Note: to get a \"standard\" Gabor patch\n% we set a grey background offset, disable normalisation, and set a\n% pre-contrast multiplier of 0.5).\n% Dimension of the region where will draw the Gabor in pixels\ngaborDimPix = windowRect(3);\n% Sigma of Gaussian  (how much to fade around the edges)\nsigma = gaborDimPix / 0;  % change the 0 value to alter the fading\nphasePerFrame = desiredfrequency*360*ifi;\nfreq = numCycles / gaborDimPix;\n\nbackgroundOffset = [0.5 0.5 0.5 0.0];\ndisableNorm = 1;\npreContrastMultiplier = 0.5;\ngabortex = CreateProceduralGabor(window, gaborDimPix, gaborDimPix, [],...\n    backgroundOffset, disableNorm, preContrastMultiplier);\n\n% Randomise the phase of the Gabors and make a properties matrix.\nfor N = 1:numel(contrasts)\npropertiesMat{1,N} = [phase, freq, sigma, contrasts(N), aspectRatio, 0, 0, 0];\nend\n\niiii = 1;\ncchoice = RandomizedTrials(iiii);\ncont2 = contrasts(cchoice);\npm = propertiesMat{1,1};\ncurtrial = 0;\n\n%%  Build up the rectangles for the pause and hold screen\nbaseRect = [0 0 screenXpixels screenYpixels];\ncenteredRect = CenterRectOnPointd(baseRect, xCenter, yCenter);\nrectColorB = [128 128 128]/255;\nrectColorG = [128 128 128]/255;\n\n%%  Finalize the trial data and orders\nstim_id = [ones(1,NT)*1];\nreward = [ones(1,NT)*1];\nmeanITI = nanmean(intervals);\nrand_idx1 = randperm(NT);\nrand_idx2 = randperm(NT);\nintervals = intervals(rand_idx2);\nstim_id = stim_id(rand_idx2);\nreward = reward(rand_idx2);\n%%  All Done!\n%  indicate that the necessary preloading of data has been completed.\nstim_loaded = 1;" ("Script Node")("NT"=w271, "BITI"=w270, "JIT"=w269, "cont"=w268, "goEXP"=w265, "minITI"=w264, "maxITI"=w263, "lambda"=w262) -> ("stim_loaded"=w276:dbl, "intervals"=w272:dbl[], "stim_id"=w273:dbl[], "reward"=w274:dbl[], "meanITI"=→"meanITI":dbl)  [unwired: 1 in, 1 out]
            "stim_loaded" <- w276
            "Timings" <- w272
            "stim_id" <- w273
            "reward" <- w274
            n253 = shared-variable "My Computer\\michelle_library.lvlib\\Timings"(w272) -> ()  [unwired: 1 in, 1 out]
            n254 = shared-variable "My Computer\\michelle_library.lvlib\\Stim_ID"(w273) -> ()  [unwired: 1 in, 1 out]
            n255 = shared-variable "My Computer\\michelle_library.lvlib\\Reward_mat"(w274) -> ()  [unwired: 1 in, 1 out]
            n256 = Equal?(x=w276, y=1.0) -> (x = y?=→"Stimuli Loaded?":bool)
          }
        }
        n257 = local read "Stimuli Loaded?"() -> (w258:bool)
      }
    }
    frame #3 {
      n258 = Get Date/Time In Seconds() -> (seconds since 1Jan1904=w283:timestamp)
      n259 = local read "Stimuli Loaded?"() -> (w278:bool)
      n260 = local read "Initialtime"() -> (w282:dbl)
      n261 = local read "Elapsed Time"() -> (w277:dbl)
      n262 = To Double Precision Float(number=w283) -> (double precision float=w280:dbl)
      n263 = shared-variable "My Computer\\michelle_library.lvlib\\InitiatedStamp"(w280) -> ()  [unwired: 1 in, 1 out]
      n264 = Subtract(x=w280, y=w282) -> (x-y=w281:dbl)
      n265 = shared-variable "My Computer\\michelle_library.lvlib\\Stim_loaded"(w278) -> ()  [unwired: 1 in, 1 out]
      n266 = Subtract(x=w277, y=w281) -> (x-y=→"Lag1":dbl)
      n267 = shared-variable "My Computer\\michelle_library.lvlib\\InitiatedLag"(w277) -> ()  [unwired: 1 in, 1 out]
    }
  }
